vi "Spindexer_Teleop.vi"(11 "Joystick_In":T1) -> ()   [LabVIEW 2019]
uses:
  Spindexer_Cluster.ctl
  Spindexer_Globals.vi
  Spindexer_mode.ctl
  Utility_VIs/Joystick_Controls.ctl
panel:
  in  "Intake":bool
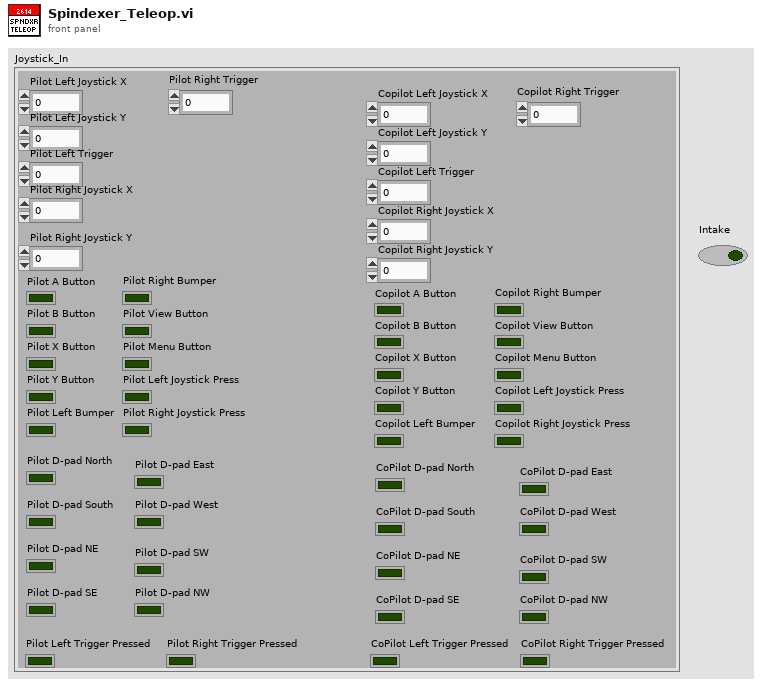
[diagram p1: front panel]
types:
  T1 = typedef "Joystick_Controls.ctl" = cluster{"Pilot Left Joystick X":dbl, "Pilot Left Joystick Y":dbl, "Pilot A Button":bool, "Pilot B Button":bool, "Pilot X Button":bool, "Pilot Y Button":bool, "Pilot Left Bumper":bool, "Pilot Right Bumper":bool, "Pilot View Button":bool, "Pilot Menu Button":bool, "Pilot Left Joystick Press":bool, "Pilot Right Joystick Press":bool, "Pilot Left Trigger":dbl, "Pilot Right Joystick X":dbl, "Pilot Right Joystick Y":dbl, "Pilot Right Trigger":dbl, "Copilot Left Joystick X":dbl, "Copilot Left Joystick Y":dbl, "Copilot A Button":bool, "Copilot B Button":bool, "Copilot X Button":bool, "Copilot Y Button":bool, "Copilot Left Bumper":bool, "Copilot Right Bumper":bool, "Copilot View Button":bool, "Copilot Menu Button":bool, "Copilot Left Joystick Press":bool, "Copilot Right Joystick Press":bool, "Copilot Left Trigger":dbl, "Copilot Right Joystick X":dbl, "Copilot Right Joystick Y":dbl, "Copilot Right Trigger":dbl, "Pilot D-pad North":bool, "Pilot D-pad South":bool, "Pilot D-pad East":bool, "Pilot D-pad West":bool, "Pilot D-pad NE ":bool, "Pilot D-pad SE":bool, "Pilot D-pad SW":bool, "Pilot D-pad NW":bool, "CoPilot D-pad North":bool, "CoPilot D-pad South":bool, "CoPilot D-pad East":bool, "CoPilot D-pad West":bool, "CoPilot D-pad NE":bool, "CoPilot D-pad SE":bool, "CoPilot D-pad SW":bool, "CoPilot D-pad NW":bool, "Pilot Left Trigger Pressed":bool, "Pilot Right Trigger Pressed":bool, "CoPilot Left Trigger Pressed":bool, "CoPilot Right Trigger Pressed":bool}
  T2 = typedef "Spindexer_Cluster.ctl" = cluster{"Throttle":dbl, "Fire?":bool, "Intake recently moved?":bool, "Mode":T3, "Sensor in position? ":bool}
  T3 = typedef "Spindexer_mode.ctl" = enum16{"No-Op", "Sensing", "Intaking", "Firing(Speed Control)", "Manual"}
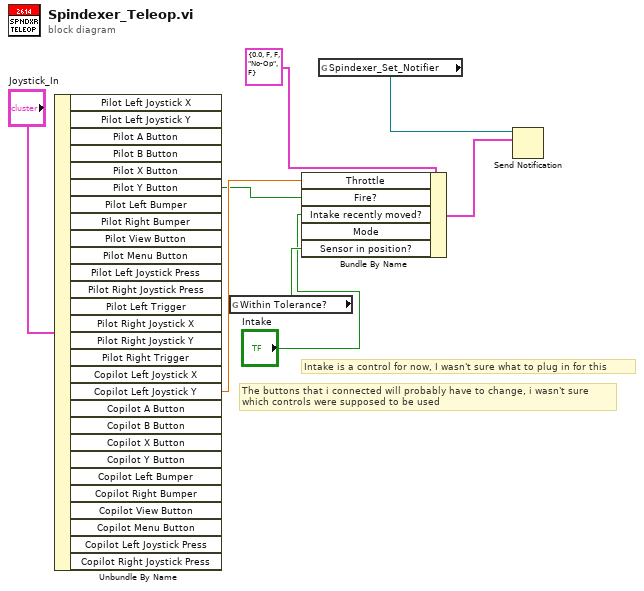
[diagram p0: block diagram]
diagram:
  # "Intake is a control for now, I wasn't sure what to plug in for this"
  # "The buttons that i connected will probably have to change, i wasn't sure\nwhich controls were supposed to be used"
  n1 = Unbundle By Name("Joystick_In") -> ("Pilot Y Button"=w4:bool, "Copilot Left Joystick Y"=w5:dbl)  [unwired: 26 out]
  n2 = global read "Spindexer_Globals.vi" "Within Tolerance?"() -> (w3:bool)
  n3 = Bundle By Name(cluster=T2 {"Throttle"=0.0, "Fire?"=FALSE, "Intake recently moved?"=FALSE, "Mode"=enum."No-Op", "Sensor in position? "=FALSE} ("Cluster"), "Throttle"=w5, "Fire?"=w4, "Intake recently moved?"="Intake", "Sensor in position?"=w3) -> (w2:T2)  [unwired: 1 in]
  n4 = global read "Spindexer_Globals.vi" "Spindexer_Set_Notifier"() -> (w7:refnum<notifier>)
  n5 = Send Notification(notification=w2, notifier=w7) -> ()  [unwired: 1 in, 2 out]
